vi "蠕动泵2动作命令 (子VI).vi"(8 "Error in":errorcluster caption="Error in (no error)", 10 "启动命令":T1(ring), 11 "仪器":enum16{"", "氨氮", "总磷", "总氮", "CODMn", "CODCr"}(ring)=enum."氨氮") -> (0 "error out":errorcluster)   [LabVIEW 2016, in "质控单元.lvlib"]
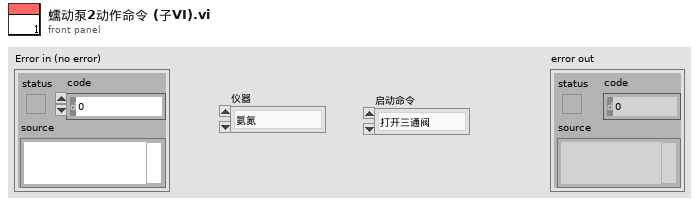
[diagram p1: front panel]
types:
  T1 = enum16{"打开三通阀", "关闭三通阀", "蠕动泵正转", "蠕动泵反转", "蠕动泵停止"}
  T2 = cluster{"仪器":enum16{"", "氨氮", "总磷", "总氮", "CODMn", "CODCr"}, "starting address":u16, "value":u16}
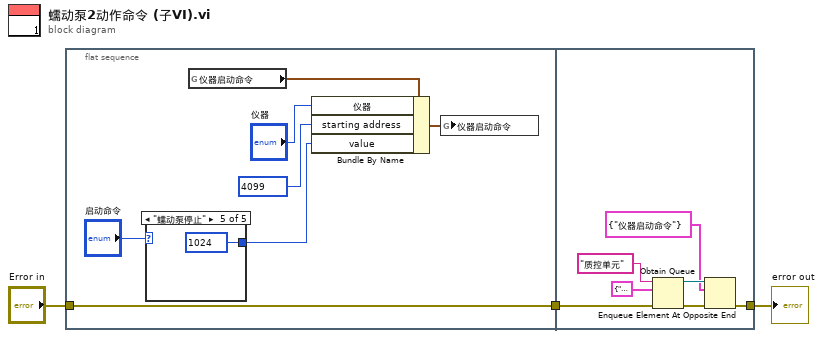
[diagram p0: block diagram]
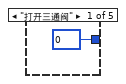
[diagram p2: hidden frame]
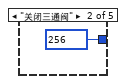
[diagram p3: hidden frame]
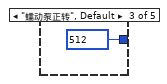
[diagram p4: hidden frame]
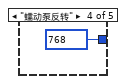
[diagram p5: hidden frame]
diagram:
  n1 = flat-sequence {
    tunnel: "Error in" -> [w8]
    tunnel: [w8] -> w3
    tunnel: w3 -> [w17]
    tunnel: [w16] -> w2
    frame #0 {
      n2 = case shown="\"蠕动泵停止\"" "启动命令" {
        tunnel: [u16 0 ("starting address") u16 256 ("starting address") u16 512 ("starting address") u16 768 ("starting address") u16 1024 ("starting address")] -> w6
        frame "打开三通阀" {
        }
        frame "关闭三通阀" {
        }
        frame "蠕动泵正转", Default {
        }
        frame "蠕动泵反转" {
        }
        frame "蠕动泵停止" {
        }
      }
      n3 = global read "质控内部交互全局.vi" "仪器启动命令"() -> (w9:T2)
      n4 = Bundle By Name(cluster=w9, "仪器"="仪器", "starting address"=u16 4099, "value"=w6) -> (w10:T2)
      n5 = global write "质控内部交互全局.vi" "仪器启动命令"(w10) -> ()
    }
    frame #1 {
      n6 = Obtain Queue(name (unnamed)="质控单元" ("名称（未命名）"), element data type=cluster{"命令":string} {"命令"="启用模块"} ("元素"), error in (no error)=w17) -> (queue out=w20:refnum<queue>, error out=w19:errorcluster)  [unwired: 2 in, 1 out]
      n7 = Enqueue Element At Opposite End(queue=w20, element=cluster{"命令":string} {"命令"="仪器启动命令"} ("元素"), error in (no error)=w19) -> (error out=w16:errorcluster)  [unwired: 1 in, 2 out]
    }
  }
  "error out" <- w2
